vi "Memory.Pointer.Duplicate.vi"(8 "error in (no error)":errorcluster, 11 "pointer in":refnum<class "Memory.Pointer.lvclass">) -> (0 "error out":errorcluster, 2 "new pointer":refnum<class "Memory.Pointer.Internal.lvclass">, 3 "pointer out":refnum<class "Memory.Pointer.lvclass">)   [LabVIEW 2016, in "Memory Manager.lvlib" / "Memory.Pointer.lvclass"]
doc: "Allocates a <b>new pointer</b> with a copy of the data referenced by the provided <b>pointer</b>."
uses:
  Memory.Pointer.lvclass
  Pointer.Internal/Memory.Pointer.Internal.lvclass
  C:/Git/SourceTree/LabVIEW-Memory-Manager/Source/Classes/Pointer/Memory.Pointer.lvclass
  Memory.Pointer.lvclass/Memory.Pointer.ctl
  Memory.Pointer.Copy All.Safe.vi
  Accessors/Set Address.vi
  Accessors/Set Size.vi
  Memory.Pointer.Copy.Safe.vi
  Memory.Pointer.Copy.Unsafe.vi
  Memory.Pointer.Parameter Check.Subset.vi
  Memory.Pointer.Parameter Check.Null Pointer.vi
  Accessors/Get Address.vi
  Memory.Pointer.Errors.vi
  Memory.Pointer.Errors.Out of Bounds.vi
  Memory.Pointer.Errors.Null Pointer.vi
  Submodules/SEH/Source/VIs/Static Error Handling.Source Buffer.Write.String.vi
  Memory.Pointer.Errors.Write Pointer Size.vi
  Memory.Pointer.Errors.Create Error.vi
  Submodules/SEH/Source/VIs/Static Error Handling.Source Buffer.Write.Numeric.Scalar.Base10.vi
  Submodules/SEH/Source/VIs/Static Error Handling.Source Buffer.Write.Numeric.Scalar.Base10 (U64).vi
  Submodules/SEH/Source/VIs/Static Error Handling.Error Cluster Constant.vi
  Submodules/SEH/Source/VIs/Static Error Handling.Error Cluster Constant (256B).vi
  Submodules/SEH/Source/VIs/Static Error Handling.Parameters.Status.Set.vi
  Submodules/SEH/Source/VIs/Static Error Handling.Parameters.Code.Set.vi
  Submodules/SEH/Source/VIs/Static Error Handling.Parameters.VI Source.Set.vi
  Constants/Memory.Constants.vi
  Constants/Memory.Constants.Library Name.vi
  Memory.Pointer.Errors.Get Info.vi
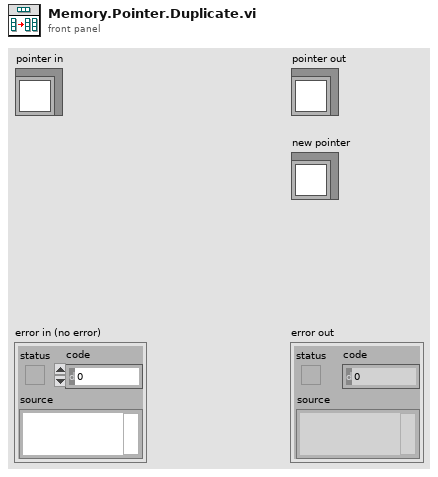
[diagram p1: front panel]
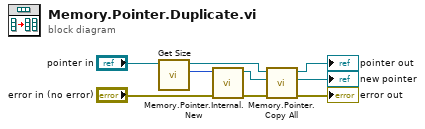
[diagram p0: block diagram]
diagram:
  n1 = call "Get Size.vi"("Pointer in"="pointer in") -> ("size"=w7:u64, "Pointer out"=w4:refnum<class "Memory.Pointer.lvclass">)  [unwired: 8 in, 1 out]
  n2 = call "Memory.Pointer.Internal.New.vi"("error in (no error)"="error in (no error)", "size"=w7) -> ("error out"=w6:errorcluster, "pointer"=w5:refnum<class "Memory.Pointer.Internal.lvclass">)  [unwired: 8 in]
  n3 = call-poly "Memory.Pointer.Copy All.vi"("error in (no error)"=w6, "dst pointer in"=w5, "src pointer in"=w4) -> ("error out"=→"error out":errorcluster, "dst pointer out"=→"new pointer":refnum<class "Memory.Pointer.Internal.lvclass">, "src pointer out"=→"pointer out":refnum<class "Memory.Pointer.lvclass">)  [unwired: 6 in]
